vi "Createxypsicsv.vi"() -> ()   [LabVIEW 2019]
uses:
  <vilib>/LabVIEW Open Source Project/Data Manipulation/Scalar/FinalStringFormatting.vi
  <vilib>/LabVIEW Open Source Project/Data Manipulation/Scalar/Get Decimal Separator.vi
  <vilib>/Utility/file.llb/Write Delimited Spreadsheet (string).vi
  <vilib>/LabVIEW Open Source Project/Data Manipulation/Scalar/OpenScalar.lvlib
panel:
  out "Psi":dbl
  in  "stop":bool
  out "X":dbl
  out "Y":dbl
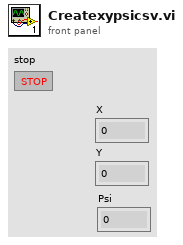
[diagram p1: front panel]
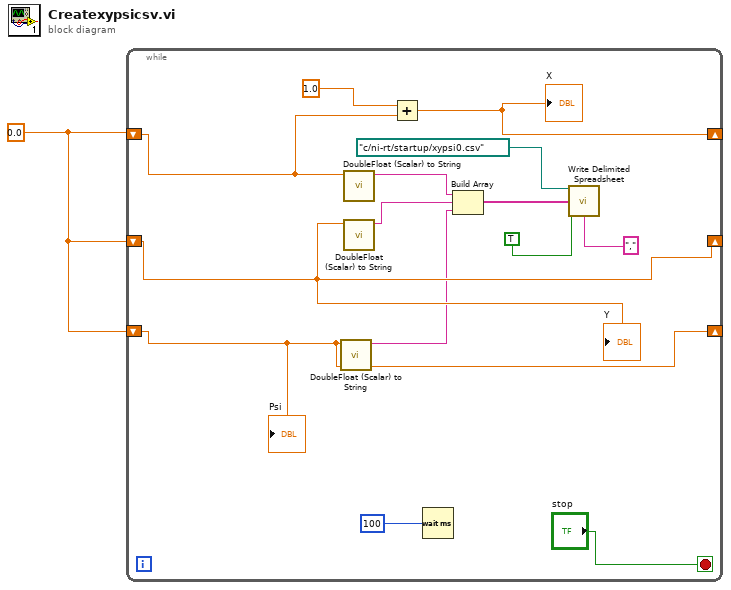
[diagram p0: block diagram]
diagram:
  w1 = 0.0
  n1 = while {
    shift-right: [w5] -> _
    shift-left: w1 -> [w6]
    shift-right: [w7] -> _
    shift-left: w1 -> [w7]
    shift-right: [w3] -> _
    shift-left: w1 -> [w3]
    stop <- "stop" stop-if-true
    n2 = call <vilib>:"DoubleFloat (Scalar) to String.vi"("Value (Double)"=w3) -> ("Value (String)"=w2:string)  [unwired: 10 in]
    n3 = call <vilib>:"DoubleFloat (Scalar) to String.vi"("Value (Double)"=w6) -> ("Value (String)"=w13:string)  [unwired: 10 in]
    n4 = call <vilib>:"DoubleFloat (Scalar) to String.vi"("Value (Double)"=w7) -> ("Value (String)"=w12:string)  [unwired: 10 in]
    n5 = Add(x=1.0, y=w6) -> (x+y=w5:dbl)
    "X" <- w5
    n6 = Wait (ms)(milliseconds to wait=u32 100) -> ()  [unwired: 1 out]
    n7 = Build Array(w13, w12, w2) -> (w9:string[])
    n8 = call-poly <vilib>:"Write Delimited Spreadsheet.vi"("file path (dialog if empty)"=path "c:/ni-rt/startup/xypsi0.csv", "1D data"=w9, "append to file? (new file:F)"=TRUE, "delimiter (\\t)"="," ("delimiter (\\t)")) -> ()  [unwired: 10 in, 2 out]
    "Y" <- w7
    "Psi" <- w3
  }
